vi "Array Average.vi"() -> ()   [LabVIEW 2025]
panel:
  out "Array Average":dbl
  in  "Input Array":dbl[](array[numeric])
  # "ME 235: Design of Microprocessor Based Mechanical Systems"
  # "Lab 2 - Array Averager"
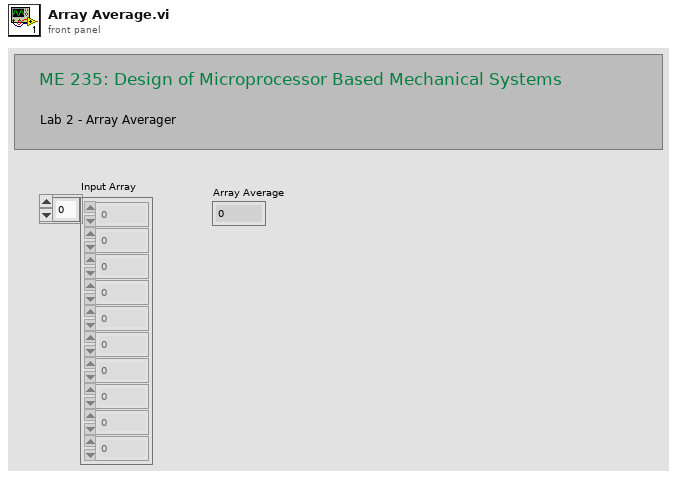
[diagram p1: front panel]
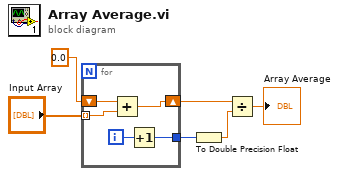
[diagram p0: block diagram]
diagram:
  n1 = for {
    tunnel: "Input Array" -> [w10] mode=indexing
    shift-right: [w8] -> w4
    shift-left: 0.0 -> [w11]
    tunnel: [w7] -> w3
    i -> [w9]
    n2 = Add(x=w11, y=w10) -> (x+y=w8:dbl)
    n3 = Increment(x=w9) -> (x+1=w7:i32)
  }
  n4 = To Double Precision Float(number=w3) -> (double precision float=w2:dbl)
  n5 = Divide(x=w4, y=w2) -> (x/y=→"Array Average":dbl)
